vi "Create Instrument SMO Name.vi"(8 "error in (no error)":errorcluster, 11 "Instrument.VoltageSource in":refnum<class "Instrument.VoltageSource.lvclass">) -> (0 "error out":errorcluster, 2 "SMO Name":string, 3 "Instrument.VoltageSource out":refnum<class "Instrument.VoltageSource.lvclass">)   [LabVIEW 2016, in "Instrument.VoltageSource.lvclass"]
uses:
  Instrument.VoltageSource.lvclass
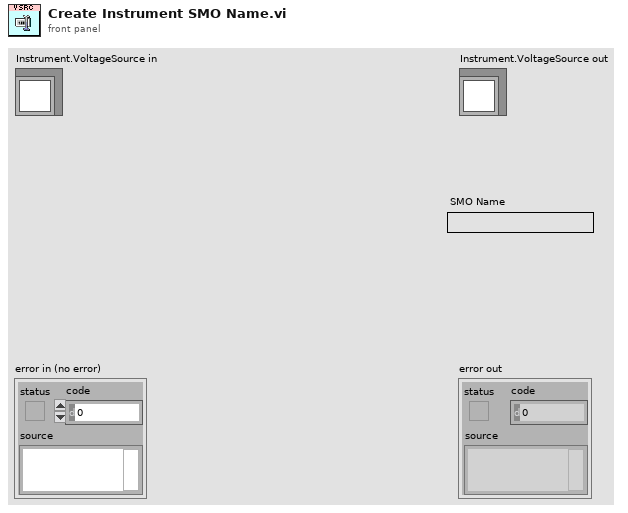
[diagram p1: front panel]
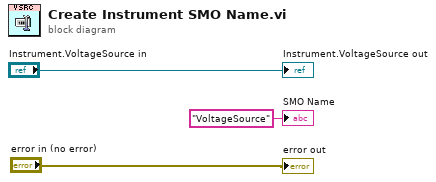
[diagram p0: block diagram]
diagram:
  "error out" <- "error in (no error)"
  "Instrument.VoltageSource out" <- "Instrument.VoltageSource in"
  "SMO Name" <- "VoltageSource" ("SMO Name")
